vi "Set Timestamp.vi"(8 "error in (no error)":errorcluster, 11 "VISA resource name":refnum<visa-resource-name>) -> (0 "error out":errorcluster, 3 "VISA resource name out":refnum<visa-resource-name>)   [LabVIEW 2015, in "Rohde&Schwarz CMXP Base.lvlib"]
doc: "This command sets a timestamp with the current system time. A timer can be started with a timeout relative to this timestamp, see SYSTem:TIME:HRTimer:ABSolute. An existing timestamp is overwritten.\n\nAttribute:\nRSCMXPBASE_ATTR_SET_TIMESTAMP\n\nRemote-control command:\nSYSTem:TIME:HRTimer:ABSolute:SET"
uses:
  <instrlib>/Rohde&Schwarz CMXP Base/Rohde&Schwarz CMXP Base.lvlib
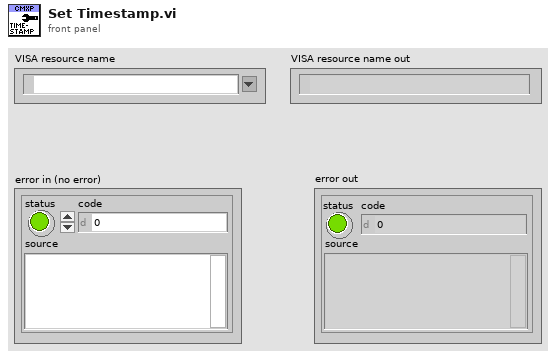
[diagram p1: front panel]
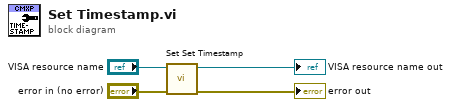
[diagram p0: block diagram]
diagram:
  n1 = call "Set Set Timestamp"("error in (no error)"="error in (no error)", "instrument handle"="VISA resource name") -> ("error out"=→"error out":errorcluster, "instrument handle out"=→"VISA resource name out":refnum<visa-resource-name>)  [unwired: 8 in]
